vi "Forward Kinematics.vi"(8 "error in (no error)":errorcluster, 11 "Grips Robot in":refnum<class "Grips Robot.lvclass">) -> (0 "error out":errorcluster, 2 "end effector transform":T1, 3 "Grips Robot out":refnum<class "Grips Robot.lvclass">)   [LabVIEW 2013, in "Grips Robot.lvclass"]
uses:
  Grips Robot.lvclass
  <vilib>/Analysis/Matrix/Datatypes/RealMatrix.ctl
  Grips Robot.lvclass/Grips Robot.ctl
  robotic_arm_labview/Kinematics/Kinematics.lvlib
  <vilib>/Analysis/Matrix/NI_Matrix.lvlib
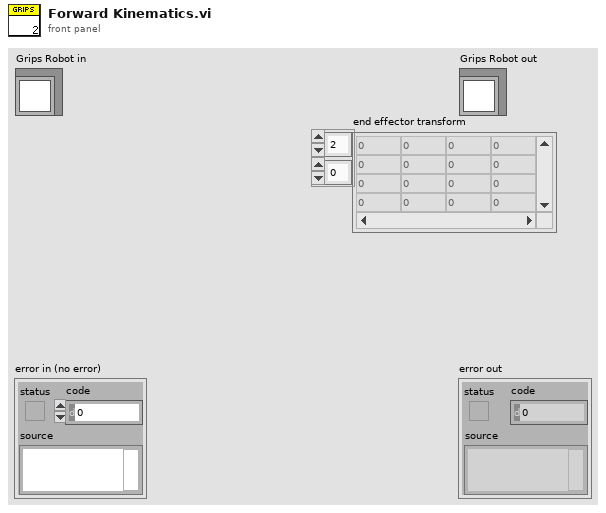
[diagram p1: front panel]
types:
  T1 = typedef "NI_Matrix.lvlib/RealMatrix.ctl" = dbl[][]
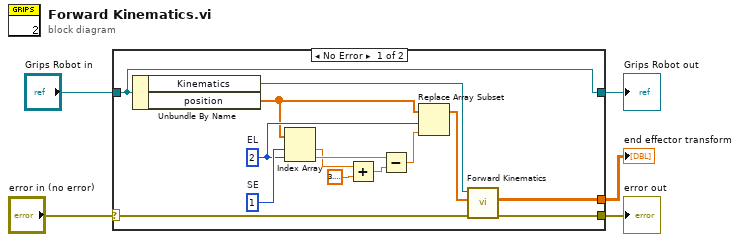
[diagram p0: block diagram]
diagram:
  n1 = case shown="No Error" "error in (no error)" {
    selector: "error in (no error)" -> [w16 w21]
    tunnel: [w17 w21] -> w4
    tunnel: [w19 w20] -> w2
    tunnel: "Grips Robot in" -> [w19 w20]
    tunnel: [w15 _] -> w1
    frame No Error {
      w13 = 1  # SE
      w12 = 2  # EL
      n2 = Unbundle By Name(w19) -> ("Kinematics"=w18:refnum<class "Robot Arm.lvclass">, "position"=w11:dbl[])
      n3 = Index Array(array=w11, index #1=w13, index #2=w12) -> (element #1=w7:dbl, element #2=w9:dbl)
      n4 = Add(x=w7, y=3.141592653589793) -> (x+y=w6:dbl)
      n5 = Subtract(x=w9, y=w6) -> (x-y=w10:dbl)
      n6 = Replace Array Subset(array=w11, new element=w10, index=w12) -> (w14:dbl[])
      n7 = call "Forward Kinematics.vi"("error in (no error)"=w16, "joint positions"=w14, "Robot Arm in"=w18) -> ("error out"=w17:errorcluster, "end effector transform"=w15:T1)  [unwired: 6 in, 1 out]
    }
    frame Error {
    }
  }
  "error out" <- w4
  "Grips Robot out" <- w2
  "end effector transform" <- w1
